vi "X Channel N.vi"(0 "EPU452 in":refnum<class "EPU452.lvclass">, 2 "Operation":string, 5 "Channel":T1, 7 "Function":string, 9 "Argument/s":string, 11 "error in (no error)":errorcluster) -> (4 "EPU452 out":refnum<class "EPU452.lvclass">, 8 "Response":string, 15 "error out":errorcluster)   [LabVIEW 2018, in "EPU452.lvclass"]
uses:
  EPU452.lvclass
  Controls/Channels.ctl
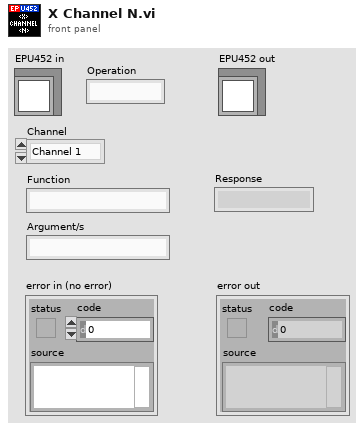
[diagram p1: front panel]
types:
  T1 = typedef "EPU452.lvclass/Channels.ctl" = enum16{"Channel 1", "Channel 2", "Channel 3", "Channel 4"}
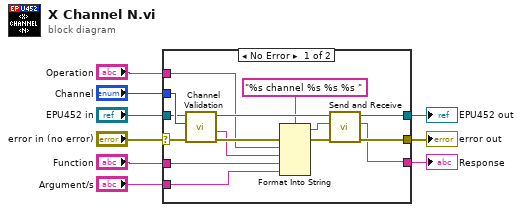
[diagram p0: block diagram]
diagram:
  n1 = case shown="No Error" "error in (no error)" {
    selector: "error in (no error)" -> [w22 w26]
    tunnel: [w18 w26] -> w8
    tunnel: [w19 w25] -> w6
    tunnel: "EPU452 in" -> [w23 w25]
    tunnel: "Channel" -> [w24 _]
    tunnel: "Function" -> [w15 _]
    tunnel: "Argument/s" -> [w14 _]
    tunnel: "Operation" -> [w17 _]
    tunnel: [w13 _] -> w1
    frame No Error {
      n2 = call "Channel Validation.vi"("error in (no error)"=w22, "Channel in"=w24, "EPU452 in"=w23) -> ("error out"=w21:errorcluster, "Channel"=w16:string, "EPU452 out"=w20:refnum<class "EPU452.lvclass">)  [unwired: 5 in, 1 out]
      n3 = Format Into String(format string="%s channel %s %s %s ", error in=w21, w17, w16, w15, w14) -> (resulting string=w10:string, error out=w11:errorcluster)  [unwired: 1 in]
      n4 = call "Send and Receive.vi"("error in (no error)"=w11, "Command"=w10, "EPU452 in"=w20) -> ("error out"=w18:errorcluster, "Response"=w13:string, "EPU452 out"=w19:refnum<class "EPU452.lvclass">)  [unwired: 6 in]
    }
    frame Error {
    }
  }
  "error out" <- w8
  "EPU452 out" <- w6
  "Response" <- w1
